vi "Get Version.vi"(8 "error in":errorcluster, 11 "dir or path to lv_proc.dll (.)":path) -> (0 "error out":errorcluster, 3 "version":string)   [LabVIEW 2013, in "LV Process library.lvlib"]
doc: "Calls lv_proc.dll function to create a new process and return pipe handle. Process is started by 'command' in 'working directory', and window is hidden if selected. Standard error pipe can be used. If directory with lv_proc.dll or path to lv_proc.dll is not specified, current application directory is used.\n\nEven if the process instance has returned exit code (i.e. process finished) the handle must be closed by proc_cleanup.vi.\n\n---\nLV Process works only with lv_proc.dll library, which is part of vipm package or should be delivered together with packed library. Placement of this dll is selected in terminal of Create Process.vi."
uses:
  LV Process library.lvlib
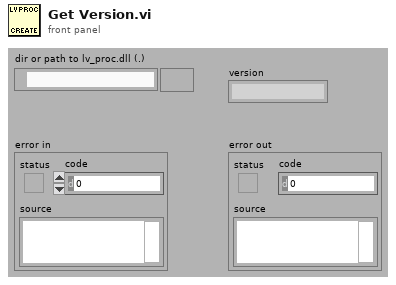
[diagram p1: front panel]
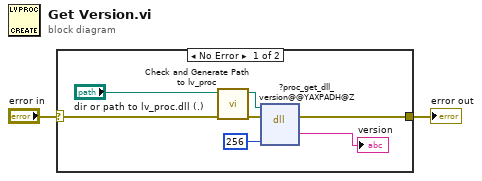
[diagram p0: block diagram]
diagram:
  n1 = case shown="No Error" "error in" {
    selector: "error in" -> [w7 w10]
    tunnel: [w3 w10] -> w1
    frame No Error {
      n2 = call "Check and Generate Path to lv_proc.vi"("error in (no error)"=w7, "dir or path to lv_proc.dll (.)"="dir or path to lv_proc.dll (.)") -> ("error out"=w6:errorcluster, "dup path"=w9:path)  [unwired: 8 in]
      n3 = dll-call lib="C:/Data/GOLPI/LV Process/lv_proc.dll" fn="?proc_get_dll_version@@YAXPADH@Z" label="proc_handle_size"(path in=w9, error in=w6, "size"=256) -> (error out=w3:errorcluster, "version"=→"version":string)  [unwired: 4 in, 1 out]
    }
    frame Error {
    }
  }
  "error out" <- w1
